vi "Plot XY.vi"() -> ()   [LabVIEW 2009]
panel:
  in  "PlotNames Array":string[](array[string])=["Temp1", "Temp2", "Temp3", "Temp4", "Temp5", "Temp6", "Temp7"]
  in  "Init Plot Cluster":T1={"Y Scale Label Left"="left", "Y Scale Label Right"="right", "X Scale Label"="Time", "Ymin Left"=0.0, "Ymax Left"=1.0, "Ymin Right"=-5.0, "Ymax Right"=5.0, "Number of Left Data"=0}
  in  "Data Array":dbl[][](array[numeric])
  in  "Time":dbl[](array[numeric])
  out "Plot":cluster{dbl[], dbl[]}[](graph)
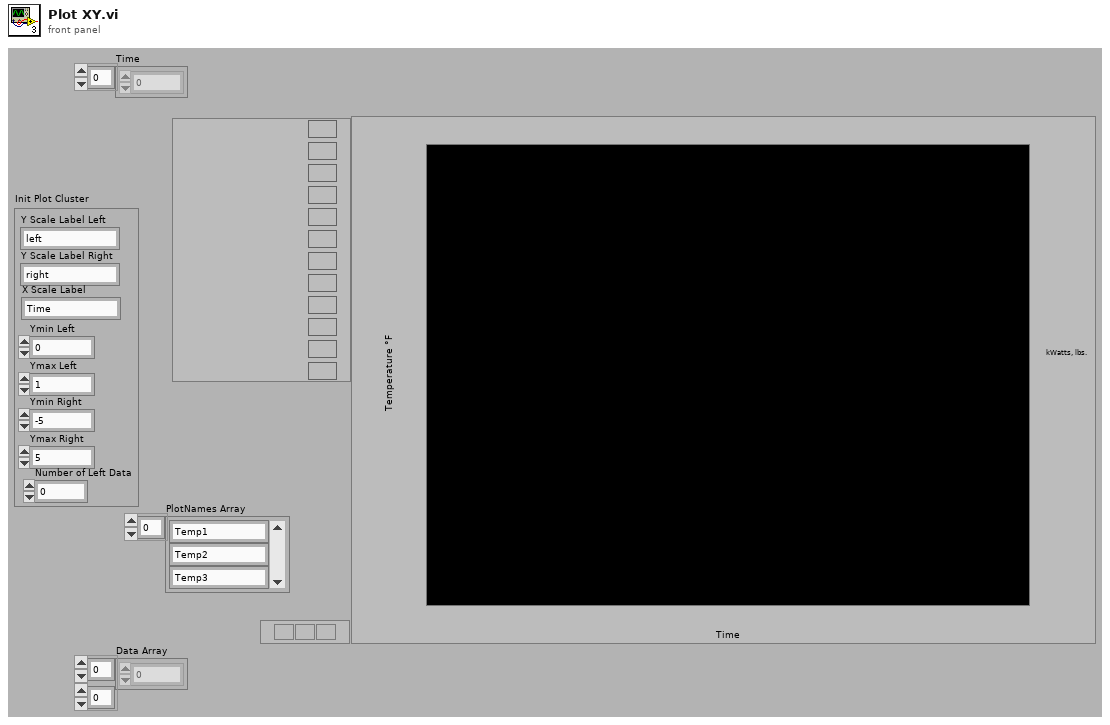
[diagram p1: front panel]
types:
  T1 = cluster{"Y Scale Label Left":string, "Y Scale Label Right":string, "X Scale Label":string, "Ymin Left":dbl, "Ymax Left":dbl, "Ymin Right":dbl, "Ymax Right":dbl, "Number of Left Data":u8}
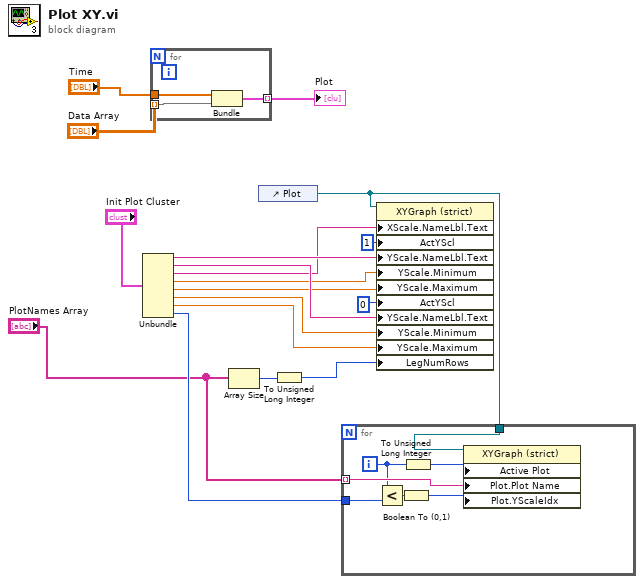
[diagram p0: block diagram]
diagram:
  n1 = Unbundle("Init Plot Cluster") -> ("Y Scale Label Left"=w10:string, "Y Scale Label Right"=w9:string, "X Scale Label"=w8:string, "Ymin Left"=w7:dbl, "Ymax Left"=w6:dbl, "Ymin Right"=w5:dbl, "Ymax Right"=w4:dbl, "Number of Left Data"=w3:u8)
  n2 = for {
    tunnel: "Time" -> [w21]
    tunnel: [w20] -> w18 mode=indexing
    tunnel: "Data Array" -> [w19] mode=indexing
    n3 = Bundle("Time"=w21, "Data Array"=w19) -> (w20:cluster{"Time":dbl[], "Data Array":dbl[]})  [unwired: 1 out]
  }
  "Plot" <- w18
  n4 = Array Size(array="PlotNames Array") -> (size(s)=w14:i32)
  n5 = control-ref of="Plot"() -> (w2:refnum<vi>)
  n6 = To Unsigned Long Integer(number=w14) -> (unsigned 32bit integer=w12:u32)
  n7 = for {
    tunnel: "PlotNames Array" -> [w28] mode=indexing
    tunnel: w3 -> [w25]
    tunnel: w2 -> [w22]
    i -> [w26]
    n8 = Less?(x=w26, y=w25) -> (x < y?=w23:bool)
    n9 = Boolean To (0,1)(Boolean=w23) -> (0, 1=w24:i16)
    n10 = To Unsigned Long Integer(number=w26) -> (unsigned 32bit integer=w27:u32)
    n11 = property on="Property Node" class="XYGraph (strict)"(reference=w22, "Active Plot"=w27, "Plot.Plot Name"=w28, "Plot.YScaleIdx"=w24) -> ()  [unwired: 1 in, 2 out]
  }
  n12 = property on="Property Node" class="XYGraph (strict)"(reference=w2, "XScale.NameLbl.Text"=w8, "ActYScl"=1 ("Active Y Scale"), "YScale.NameLbl.Text"=w10, "YScale.Minimum"=w7, "YScale.Maximum"=w6, "ActYScl"=0 ("Active Y Scale"), "YScale.NameLbl.Text"=w9, "YScale.Minimum"=w5, "YScale.Maximum"=w4, "LegNumRows"=w12) -> ()  [unwired: 1 in, 2 out]
